vi "Prober_MoveToXYZTheta.vi"(6 "Theta location [mdeg]":string="none", 7 "SemiProbe in":refnum<class "SemiProbe.lvclass">, 8 "error in (no error)":errorcluster, 9 "Z location [µm]":string="none", 10 "Y location [µm]":string="none", 11 "X location [µm]":string="none") -> (0 "error out":errorcluster, 2 "String":string, 3 "SemiProbe out":refnum<class "SemiProbe.lvclass">)   [LabVIEW 2019, in "SemiProbe.lvclass"]
uses:
  SemiProbe.lvclass
panel:
  out "t1 2":u32
  out "t1":u32
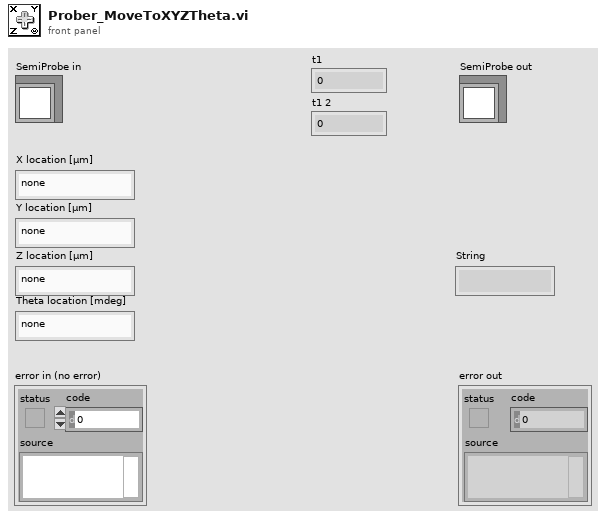
[diagram p1: front panel]
types:
  T1 = cluster{"SP Load Less Than Thr?":bool, "SP Load Threshold (um)":dbl, "SP Current Location":cluster{"X (um)":ext, "Y (um)":ext, "Z (um)":ext, "T (degree)":ext}, "SP Chuck Speeds":cluster{"XY Speed (10-100%)":dbl, "Z Speed (10-100%)":dbl, "T Speed (10-100%)":dbl}, "Manual Step Parameters":cluster{"Step in X":bool, "X S-Speed [µm/step]":sgl, "Step in Y":bool, "Y S-Speed [µm/step]":sgl, "Step in Z":bool, "Z S-Speed [µm/step]":sgl, "Step in T":bool, "T S-Speed [mdegree/step]":sgl, "X Increase":bool, "Y Increase?":bool, "Z Increase?":bool, "T Increase?":bool}, "Z Stepper":cluster{"UP/DOWN":bool, "UP/DOWN Speed [µm/step]":i32, "SP Z Step":bool}, "Z Heights Set":bool, "SP Contact Search":cluster{"Contact Circuit":enum16{"12", "1", "2"}, "Speed [1000-10000]":sgl, "Start Height [µm]":sgl, "Search Band [µm]":sgl, "Overdrive [µm]":sgl}, "Separation Distance [µm]":u32, "Contact Height [µm]":u32, "Use Overdrive?":bool, "Touchdown method":enum16{"no feedback", "Arduino edgesense", "SP contact circuit"}, "Arduino Edgesense params":cluster{"touchdown height [µm]":i32, "search band [µm]":u32, "speed [µm/step]":u32, "overdrive [µm]":u32}}
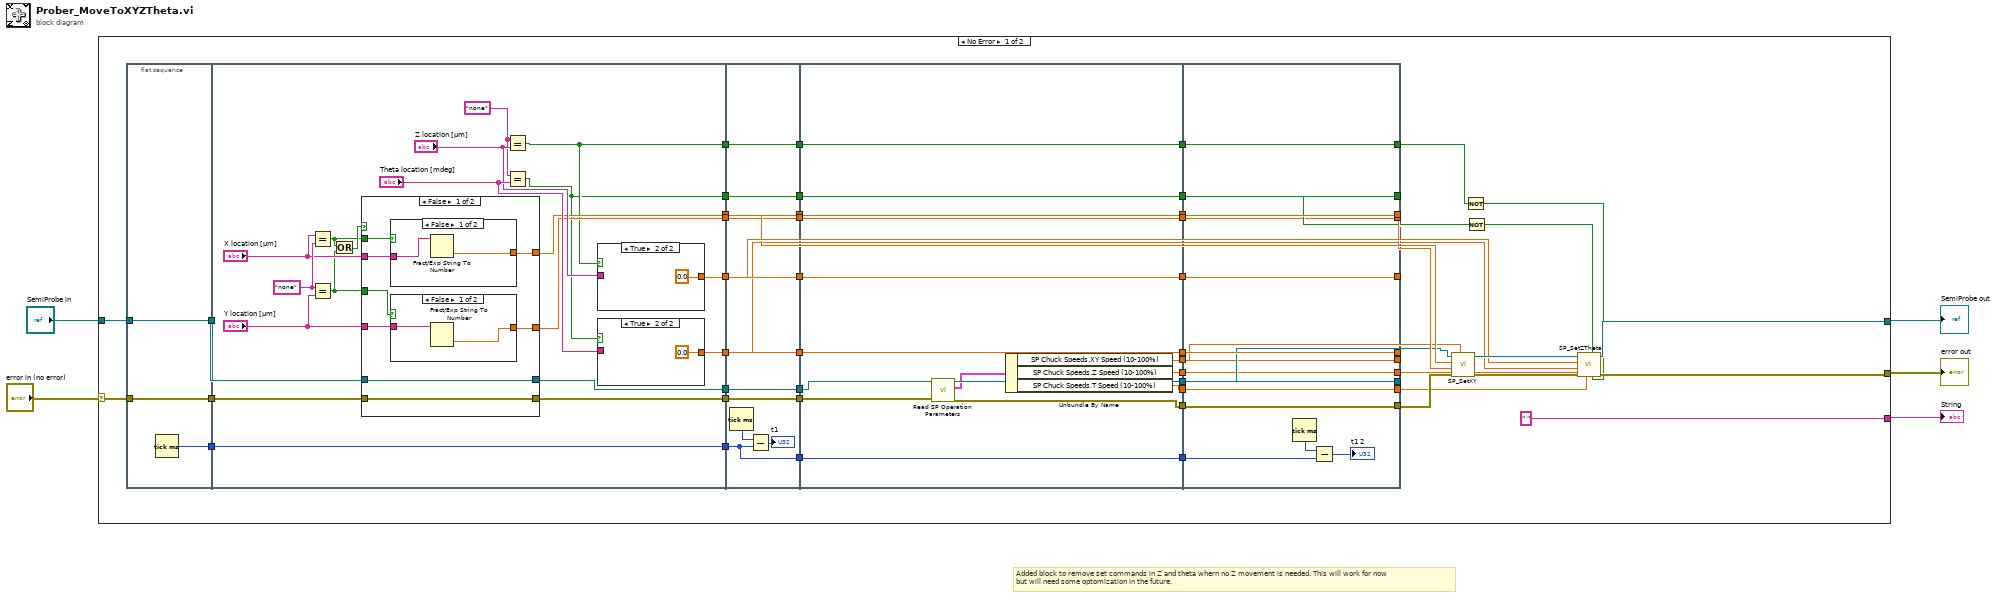
[diagram p0: block diagram]
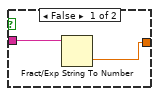
[diagram p2: hidden frame]
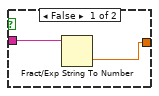
[diagram p3: hidden frame]
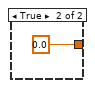
[diagram p4: hidden frame]
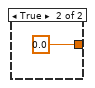
[diagram p5: hidden frame]
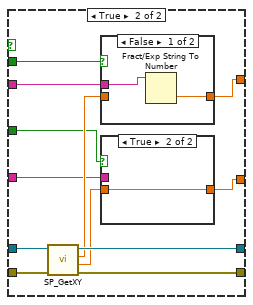
[diagram p6: hidden frame]
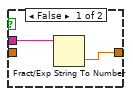
[diagram p7: hidden frame]
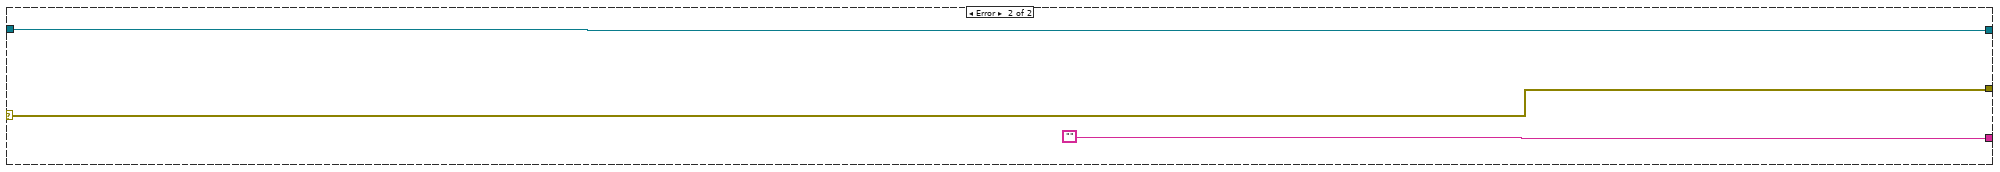
[diagram p9: hidden frame]
diagram:
  # "Added block to remove set commands in Z and theta whern no Z movement is needed. This will work for now \nbut will need some optomization in the future."
  n1 = case shown="No Error" "error in (no error)" {
    selector: "error in (no error)" -> [w56 w162]
    tunnel: "SemiProbe in" -> [w55 w161]
    tunnel: [w54 w162] -> w3
    tunnel: [w53 w161] -> w2
    tunnel: [" " ""] -> w1
    frame No Error {
      n2 = flat-sequence {
        tunnel: w55 -> [w60]
        tunnel: w56 -> [w61]
        tunnel: [w61] -> w43
        tunnel: [w60] -> w42
        tunnel: [w59] -> w32
        tunnel: w43 -> [w81]
        tunnel: w42 -> [w80]
        tunnel: [w79] -> w41
        tunnel: [w78] -> w40
        tunnel: [w70] -> w39
        tunnel: [w69] -> w38
        tunnel: [w68] -> w37
        tunnel: [w65] -> w36
        tunnel: [w64] -> w35
        tunnel: [w63] -> w34
        tunnel: [w62] -> w33
        tunnel: w32 -> [w62]
        tunnel: w41 -> [w130]
        tunnel: w40 -> [w129]
        tunnel: w39 -> [w128]
        tunnel: w38 -> [w127]
        tunnel: w37 -> [w126]
        tunnel: w36 -> [w125]
        tunnel: w35 -> [w124]
        tunnel: w34 -> [w123]
        tunnel: w33 -> [w120]
        tunnel: [w130] -> w31
        tunnel: [w129] -> w30
        tunnel: [w128] -> w29
        tunnel: [w127] -> w28
        tunnel: [w126] -> w27
        tunnel: [w125] -> w26
        tunnel: [w124] -> w25
        tunnel: [w123] -> w24
        tunnel: [w120] -> w6
        tunnel: w31 -> [w138]
        tunnel: w30 -> [w139]
        tunnel: w29 -> [w145]
        tunnel: w28 -> [w144]
        tunnel: w27 -> [w143]
        tunnel: w26 -> [w142]
        tunnel: w25 -> [w141]
        tunnel: w24 -> [w140]
        tunnel: [w145] -> w18
        tunnel: [w144] -> w17
        tunnel: [w143] -> w16
        tunnel: [w142] -> w15
        tunnel: [w141] -> w14
        tunnel: [w140] -> w13
        tunnel: [w137] -> w12
        tunnel: [w136] -> w11
        tunnel: [w134] -> w10
        tunnel: [w133] -> w9
        tunnel: [w132] -> w8
        tunnel: [w131] -> w7
        tunnel: w6 -> [w131]
        tunnel: [w149] -> w19
        tunnel: [w150] -> w20
        tunnel: [w151] -> w21
        tunnel: [w152] -> w22
        tunnel: [w153] -> w23
        tunnel: [w154] -> w45
        tunnel: [w155] -> w47
        tunnel: [w156] -> w48
        tunnel: [w157] -> w50
        tunnel: [w158] -> w51
        tunnel: [w159] -> w52
        tunnel: w18 -> [w159]
        tunnel: w17 -> [w158]
        tunnel: w16 -> [w157]
        tunnel: w15 -> [w156]
        tunnel: w14 -> [w155]
        tunnel: w13 -> [w154]
        tunnel: w12 -> [w153]
        tunnel: w11 -> [w152]
        tunnel: w10 -> [w151]
        tunnel: w9 -> [w150]
        tunnel: w8 -> [w149]
        tunnel: w7 -> [w146]
        frame #0 {
          n3 = Tick Count (ms)() -> (millisecond timer value=w59:u32)
        }
        frame #1 {
          w71 = "none"
          w76 = "none"
          n4 = Equal?(x="X location [µm]", y=w76) -> (x = y?=w67:bool)
          n5 = Equal?(x=w76, y="Y location [µm]") -> (x = y?=w66:bool)
          n6 = Or(x=w67, y=w66) -> (x .or. y?=w77:bool)
          n7 = case shown="False" w77 {
            tunnel: w81 -> [w93 w113]
            tunnel: w80 -> [w92 w112]
            tunnel: [w93 w111] -> w78
            tunnel: [w92 w110] -> w79
            tunnel: "X location [µm]" -> [w95 w107]
            tunnel: "Y location [µm]" -> [w94 w106]
            tunnel: [w91 w105] -> w68
            tunnel: [w90 w104] -> w69
            tunnel: w67 -> [w89 w103]
            tunnel: w66 -> [w88 w102]
            frame False {
              n8 = case shown="False" w89 {
                tunnel: w95 -> [w97 _]
                tunnel: [w96 0.0] -> w90
                frame False {
                  n9 = Fract/Exp String To Number(string=w97) -> (number=w96:dbl)  [unwired: 3 in, 1 out]
                }
                frame True {
                }
              }
              n10 = case shown="False" w88 {
                tunnel: w94 -> [w100 _]
                tunnel: [w99 0.0] -> w91
                frame False {
                  n11 = Fract/Exp String To Number(string=w100) -> (number=w99:dbl)  [unwired: 3 in, 1 out]
                }
                frame True {
                }
              }
            }
            frame True {
              n12 = call-dynamic "SP_GetXY.vi"("error in (no error)"=w113, "SemiProbe in"=w112) -> ("error out"=w111:errorcluster, "Y out"=w109:dbl, "X out"=w108:dbl, "SemiProbe out"=w110:refnum<class "SemiProbe.lvclass">)  [unwired: 6 in]
              n13 = case shown="False" w103 {
                tunnel: w108 -> [_ w119]
                tunnel: w107 -> [w118 _]
                tunnel: [w117 w119] -> w104
                frame False {
                  n14 = Fract/Exp String To Number(string=w118) -> (number=w117:dbl)  [unwired: 3 in, 1 out]
                }
                frame True {
                }
              }
              n15 = case shown="True" w102 {
                tunnel: w109 -> [_ w116]
                tunnel: [w115 w116] -> w105
                tunnel: w106 -> [w114 _]
                frame False {
                  n16 = Fract/Exp String To Number(string=w114) -> (number=w115:dbl)  [unwired: 3 in, 1 out]
                }
                frame True {
                }
              }
            }
          }
          n17 = Equal?(x=w71, y="Z location [µm]") -> (x = y?=w64:bool)
          n18 = Equal?(x=w71, y="Theta location [mdeg]") -> (x = y?=w63:bool)
          n19 = case shown="True" w64 {
            tunnel: "Z location [µm]" -> [w86 _]
            tunnel: [w85 0.0] -> w70
            frame False {
              n20 = Fract/Exp String To Number(string=w86) -> (number=w85:dbl)  [unwired: 3 in, 1 out]
            }
            frame True {
            }
          }
          n21 = case shown="True" w63 {
            tunnel: "Theta location [mdeg]" -> [w83 _]
            tunnel: [w82 0.0] -> w65
            frame False {
              n22 = Fract/Exp String To Number(string=w83) -> (number=w82:dbl)  [unwired: 3 in, 1 out]
            }
            frame True {
            }
          }
        }
        frame #2 {
          n23 = Tick Count (ms)() -> (millisecond timer value=w122:u32)
          n24 = Subtract(x=w122, y=w120) -> (x-y=→"t1":u32)
        }
        frame #3 {
          n25 = call-dynamic "Read SP Operation Parameters.vi"("error in (no error)"=w139, "SemiProbe in"=w138) -> ("error out"=w137:errorcluster, "SP Operation Parameters"=w135:T1, "SemiProbe out"=w136:refnum<class "SemiProbe.lvclass">)  [unwired: 7 in]
          n26 = Unbundle By Name(w135) -> ("SP Chuck Speeds.XY Speed (10-100%)"=w134:dbl, "SP Chuck Speeds.Z Speed (10-100%)"=w133:dbl, "SP Chuck Speeds.T Speed (10-100%)"=w132:dbl)
        }
        frame #4 {
          n27 = Tick Count (ms)() -> (millisecond timer value=w148:u32)
          n28 = Subtract(x=w148, y=w146) -> (x-y=→"t1 2":u32)
        }
      }
      n29 = call-dynamic "SP_SetXY.vi"("XY Speed (10-100%)"=w21, "error in (no error)"=w23, "Y in um"=w50, "X in um"=w51, "SemiProbe in"=w22) -> ("error out"=w58:errorcluster, "SemiProbe out"=w57:refnum<class "SemiProbe.lvclass">)  [unwired: 5 in]
      n30 = Not(x=w47) -> (.not. x?=w46:bool)
      n31 = Not(x=w45) -> (.not. x?=w44:bool)
      n32 = call-dynamic "SP_SetZTheta.vi"("Move Z?"=w46, "Move Theta?"=w44, "Theta Speed (10-100%)"=w19, "Z Speed (10-100%)"=w20, "error in (no error)"=w58, "Theta in mdeg"=w48, "Z in um"=w52, "SemiProbe in"=w57) -> ("error out"=w54:errorcluster, "SemiProbe out"=w53:refnum<class "SemiProbe.lvclass">)  [unwired: 2 in]
    }
    frame Error {
    }
  }
  "error out" <- w3
  "SemiProbe out" <- w2
  "String" <- w1
